vi "Array to Time Stamp.vi"(7 "6 Byte Times Stamp":u8[](array[numeric])) -> (8 "Seconds as DBL":dbl, 14 "Time Stamp Control":timestamp)   [LabVIEW 2017]
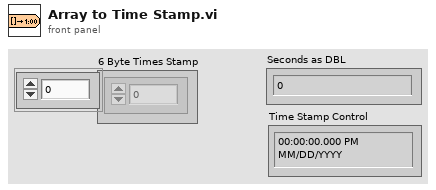
[diagram p1: front panel]
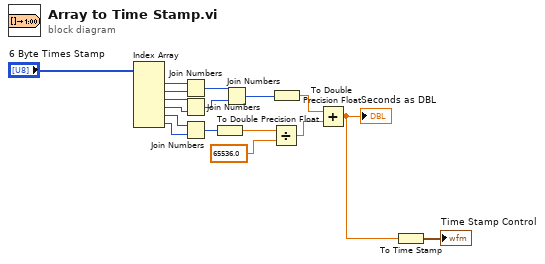
[diagram p0: block diagram]
diagram:
  n1 = Index Array(array="6 Byte Times Stamp") -> (element #1=w15:u8, element #2=w16:u8, element #3=w14:u8, element #4=w13:u8, element #5=w9:u8, element #6=w8:u8)  [unwired: 6 in]
  n2 = Join Numbers(hi=w15, lo=w16) -> ((hi.lo)=w12:u16)
  n3 = Join Numbers(hi=w14, lo=w13) -> ((hi.lo)=w10:u16)
  n4 = Join Numbers(hi=w9, lo=w8) -> ((hi.lo)=w7:u16)
  n5 = To Double Precision Float(number=w7) -> (double precision float=w6:dbl)
  n6 = Join Numbers(hi=w12, lo=w10) -> ((hi.lo)=w11:u32)
  n7 = Divide(x=w6, y=65536.0) -> (x/y=w4:dbl)
  n8 = To Double Precision Float(number=w11) -> (double precision float=w3:dbl)
  n9 = Add(x=w3, y=w4) -> (x+y=w2:dbl)
  "Seconds as DBL" <- w2
  n10 = To Time Stamp(1:w2) -> (0:→"Time Stamp Control":timestamp)
